vi "Download Attachment.vi"(6 "Authorization":T1[](array[typedef]), 8 "error in (no error)":errorcluster, 10 "Task GID":string) -> (0 "error out":errorcluster)   [LabVIEW 2016]
uses:
  <vilib>/addons/_JKI.lib/REST Client/classes/REST Client/HTTP Header.ctl
  <vilib>/addons/_JKI.lib/REST Client/classes/REST Client/REST Client.lvclass
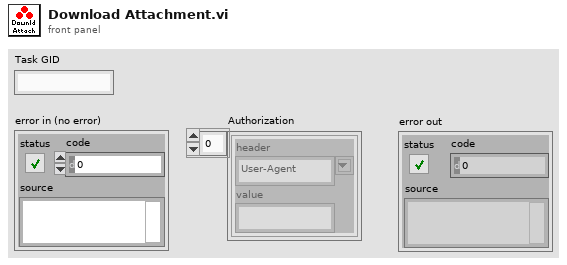
[diagram p1: front panel]
types:
  T1 = typedef "REST Client.lvlib/REST Client.lvclass/HTTP Header.ctl" = cluster{"header":string, "value":string}
  T2 = cluster{"gid":string, "resource_type":string, "name":string}[]
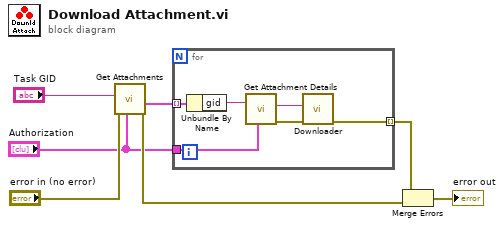
[diagram p0: block diagram]
diagram:
  n1 = call "Get Attachments.vi"("Authorization"="Authorization", "error in (no error)"="error in (no error)", "Task GID"="Task GID") -> ("error out"=w4:errorcluster, "data"=w6:T2)  [unwired: 7 in]
  n2 = for {
    tunnel: w6 -> [w13] mode=indexing
    tunnel: [w11] -> w3 mode=indexing
    tunnel: "Authorization" -> [w8]
    n3 = Unbundle By Name(w13) -> ("gid"=w12:string)
    n4 = call "Get Attachment Details.vi"("Authorization"=w8, "Attachment GID"=w12) -> ("error out"=w10:errorcluster, "download url"=w9:string)  [unwired: 7 in, 1 out]
    n5 = call "Downloader.vi"("error in"=w10, "Source URL"=w9) -> ("error out"=w11:errorcluster)  [unwired: 9 in]
  }
  n6 = Merge Errors(w3, w4) -> (→"error out":errorcluster)
